vi "Arrange SubPanels.vi"(7 "SubPanels":refnum<vi>[](array[refnum]), 8 "error in (no error)":errorcluster, 9 "Module List":string[](array[string]), 10 "上窗格":refnum<vi>, 11 "VI Reference":refnum<vi>) -> (0 "error out":errorcluster)   [LabVIEW 2020, in "Group Interface.lvlib"]
uses:
  Group Interface.lvlib
  <vilib>/Utility/miscctls.llb/LVPositionTypeDef.ctl
  <vilib>/Utility/miscctls.llb/LVBoundsTypeDef.ctl
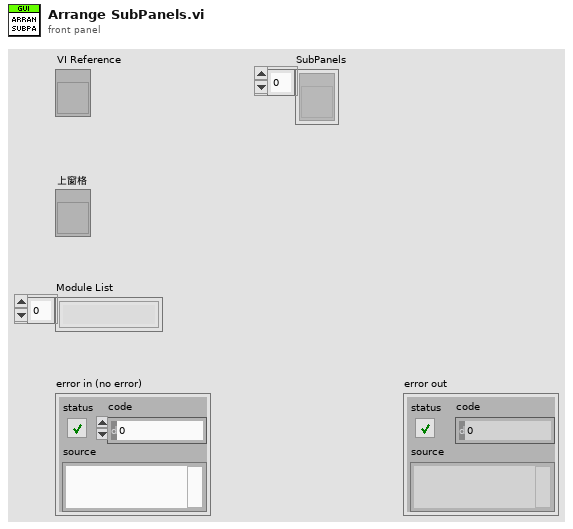
[diagram p1: front panel]
types:
  T1 = typedef "LVPositionTypeDef.ctl" = cluster{"Left":i32, "Top":i32}
  T2 = typedef "LVBoundsTypeDef.ctl" = cluster{"Width":u32, "Height":u32}
  T3 = typedef "LVRectTypeDef.ctl" = cluster{"Left":i16, "Top":i16, "Right":i16, "Bottom":i16}
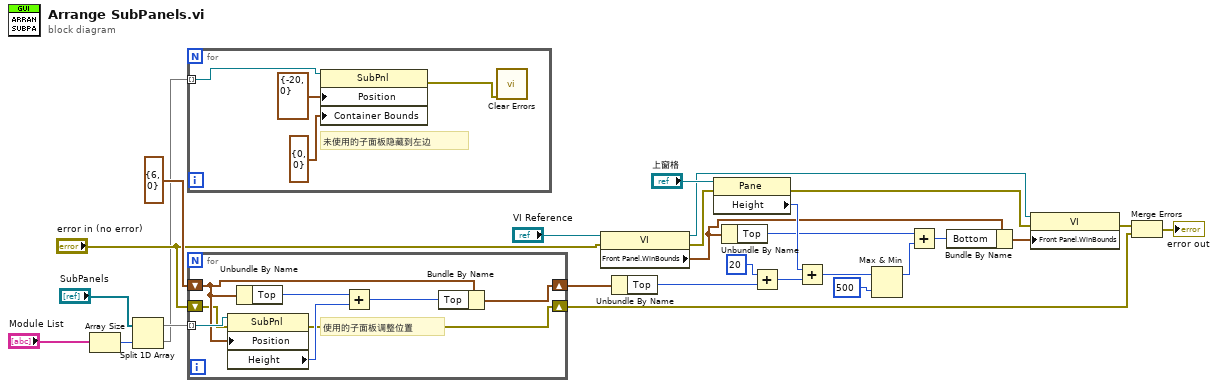
[diagram p0: block diagram]
diagram:
  n1 = Array Size(array="Module List") -> (size(s)=w25:i32)
  n2 = Split 1D Array(array="SubPanels", index=w25) -> (first subarray=w24:refnum<vi>[], second subarray=w1:refnum<vi>[])
  n3 = for {
    tunnel: w1 -> [w31] mode=indexing
    # "未使用的子面板隐藏到左边"
    n4 = property class="SubPnl"(reference=w31, "Position"=T1 {"Left"=-20, "Top"=0}, "Container Bounds"=T2 {"Width"=0, "Height"=0}) -> (error out=w28:errorcluster)  [unwired: 1 in, 1 out]
    n5 = call <vilib>:"Clear Errors.vi"("error in (no error)"=w28) -> ()  [unwired: 5 in, 2 out]
  }
  n6 = for {
    tunnel: w24 -> [w39] mode=indexing
    shift-right: [w34] -> w19
    shift-left: T1 {"Left"=6, "Top"=0} ("Position") -> [w36]
    shift-right: [w32] -> w6
    shift-left: "error in (no error)" -> [w33]
    # "使用的子面板调整位置"
    n7 = property class="SubPnl"(reference=w39, error in=w33, "Position"=w36) -> (error out=w32:errorcluster, "Height"=w38:u32)  [unwired: 1 out]
    n8 = Unbundle By Name(w36) -> ("Top"=w37:i32)
    n9 = Add(x=w37, y=w38) -> (x+y=w35:u32)
    n10 = Bundle By Name(cluster=w36, "Top"=w35) -> (w34:T1)
  }
  n11 = property class="VI"(reference="VI Reference", error in="error in (no error)") -> (reference out=w20:refnum<vi>, error out=w3:errorcluster, "Front Panel.WinBounds"=w10:T3)
  n12 = Unbundle By Name(w19) -> ("Top"=w18:i32)
  n13 = property class="Pane"(reference="上窗格", error in=w3) -> (error out=w2:errorcluster, "Height"=w15:u32)  [unwired: 1 out]
  n14 = Unbundle By Name(w10) -> ("Top"=w14:i16)
  n15 = Add(x=20, y=w18) -> (x+y=w16:i32)
  n16 = Add(x=w15, y=w16) -> (x+y=w13:u32)
  n17 = Max & Min(x=w13, y=u32 500) -> (max(x,y)=w11:u32)  [unwired: 1 out]
  n18 = Add(x=w14, y=w11) -> (x+y=w9:u32)
  n19 = Bundle By Name(cluster=w10, "Bottom"=w9) -> (w8:T3)
  n20 = property class="VI"(reference=w20, error in=w2, "Front Panel.WinBounds"=w8) -> (error out=w7:errorcluster)  [unwired: 1 out]
  n21 = Merge Errors(w7, w6) -> (→"error out":errorcluster)
